vi "Teleop.vi"(10 "Match Info":T1={"Autonomous Elapsed Seconds"=0.0, "TeleOp Elapsed Seconds"=0.0, "Disabled Elapsed Seconds"=0.0, "Visited Autonomous"=FALSE, "Visited TeleOp"=FALSE, "Visited Disabled"=FALSE, "Autonomous Settings"={"Autonomous Style"=enum."Independent", "VI Refnum"=refnum}}, 11 "Call Context":T2) -> ()   [LabVIEW 2013]
doc: "This VI is called for each TeleOp packet received from the DS where the robot is not disabled. It is often used to read from the joysticks and update I/O or to update setpoints for timed control loops. It should complete and return within 20 milliseconds or it may miss DS packets."
uses:
  <vilib>/Rock Robotics/WPI/DriverStation/WPI_DriverStationDerivedRobotMode.ctl
  <vilib>/Rock Robotics/WPI/DriverStation/WPI_DriverStationMatch Info.ctl
  Robot Global Data.vi
  <vilib>/Rock Robotics/WPI/Joystick/WPI_JoystickGetSetRefNum.vi
panel:
  in  "HarvSpeed":dbl=0.5
  out "Distance 2":dbl
  out "Distance":dbl
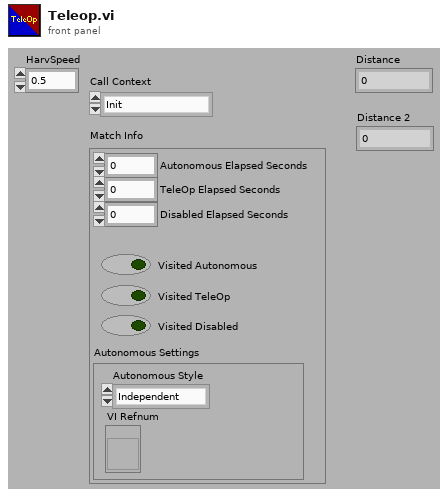
[diagram p1: front panel]
types:
  T1 = typedef "WPI_DriverStationMatch Info.ctl" = cluster{"Autonomous Elapsed Seconds":dbl, "TeleOp Elapsed Seconds":dbl, "Disabled Elapsed Seconds":dbl, "Visited Autonomous":bool, "Visited TeleOp":bool, "Visited Disabled":bool, "Autonomous Settings":cluster{"Autonomous Style":enum16{"Iterative", "Independent"}, "VI Refnum":refnum<vi>}}
  T2 = typedef "WPI_DriverStationDerivedRobotMode.ctl" = enum16{"Init", "Execute", "Stop"}
  T3 = typedef "WPI_JoystickDevRef.ctl" = cluster{"Device":T4}
  T4 = typedef "WPI_JoystickDeviceEnum.ctl" = enum16{"USB 1", "USB 2", "USB 3", "USB 4", "Kinect 1", "Kinect 2"}
  T5 = cluster{"axis 1 (x)":dbl, "axis 2 (y)":dbl, "axis 3 (throttle)":dbl, "axis 4":dbl, "axis 5":dbl, "axis 6":dbl}
  T6 = typedef "WPI_MotorControlDeviceRef.ctl" = cluster{"DeviceStatus":errorcluster, "Type":enum16{"PWM", "CAN"}, "PWM":cluster{"Digital Module":T7, "PWM Channel":T8, "DeadBand":T9}, "CAN":cluster{"Device Number":u8, "Control Mode":T10, "Semaphore":T11, "Max Vout":dbl}, "Invert":bool, "TransformRef":T12, "InvTransformRef":T12}
  T7 = typedef "FPGA_TypedefDigitalModule.ctl" = enum16{"Digital Module 1", "Digital Module 2"}
  T8 = typedef "FPGA_DIOPWMChannel.ctl" = enum8{"PWM 1", "PWM 2", "PWM 3", "PWM 4", "PWM 5", "PWM 6", "PWM 7", "PWM 8", "PWM 9", "PWM 10", "Invalid"}
  T9 = typedef "WPI_PWMDeadband.ctl" = cluster{"Name":string, "maxPositivePwm":i32, "minPositivePwm":i32, "centerPwm":i32, "maxNegativePwm":i32, "minNegativePwm":i32, "angularRange":u16}
  T10 = typedef "WPI_CANJaguar_ControlMode.ctl" = enum8{"Percent VBus", "Current", "Speed", "Position", "Voltage"}
  T11 = typedef "Semaphore RefNum" = refnum<k1>
  T12 = typedef "WPI_PWMTransform_ConPane.ctl" = refnum<vi>
  T13 = typedef "WPI_EncoderDevRef.ctl" = cluster{"DevStatus":errorcluster, "EncoderIndex":T14, "CounterIndex":T15, "DistancePerCount":dbl, "Decoding Type":T16}
  T14 = typedef "FPGA_EncoderIdx.ctl" = enum8{"Enc 0", "Enc 1", "Enc 2", "Enc 3", "Invalid"}
  T15 = typedef "FPGA_CounterCtrSystemIndex.ctl" = enum8{"Ctr 0", "Ctr 1", "Ctr 2", "Ctr 3", "Ctr 4", "Ctr 5", "Ctr 6", "Ctr 7", "Invalid"}
  T16 = typedef "WPI_EncoderType.ctl" = enum16{"1x", "2x", "4x"}
  T17 = typedef "WPI_JoystickButtonState.ctl" = cluster{"Button 1":bool, "Button 2":bool, "Button 3":bool, "Button 4":bool, "Button 5":bool, "Button 6":bool, "Button 7":bool, "Button 8":bool, "Button 9":bool, "Button 10":bool, "Button 11":bool, "Button 12":bool}
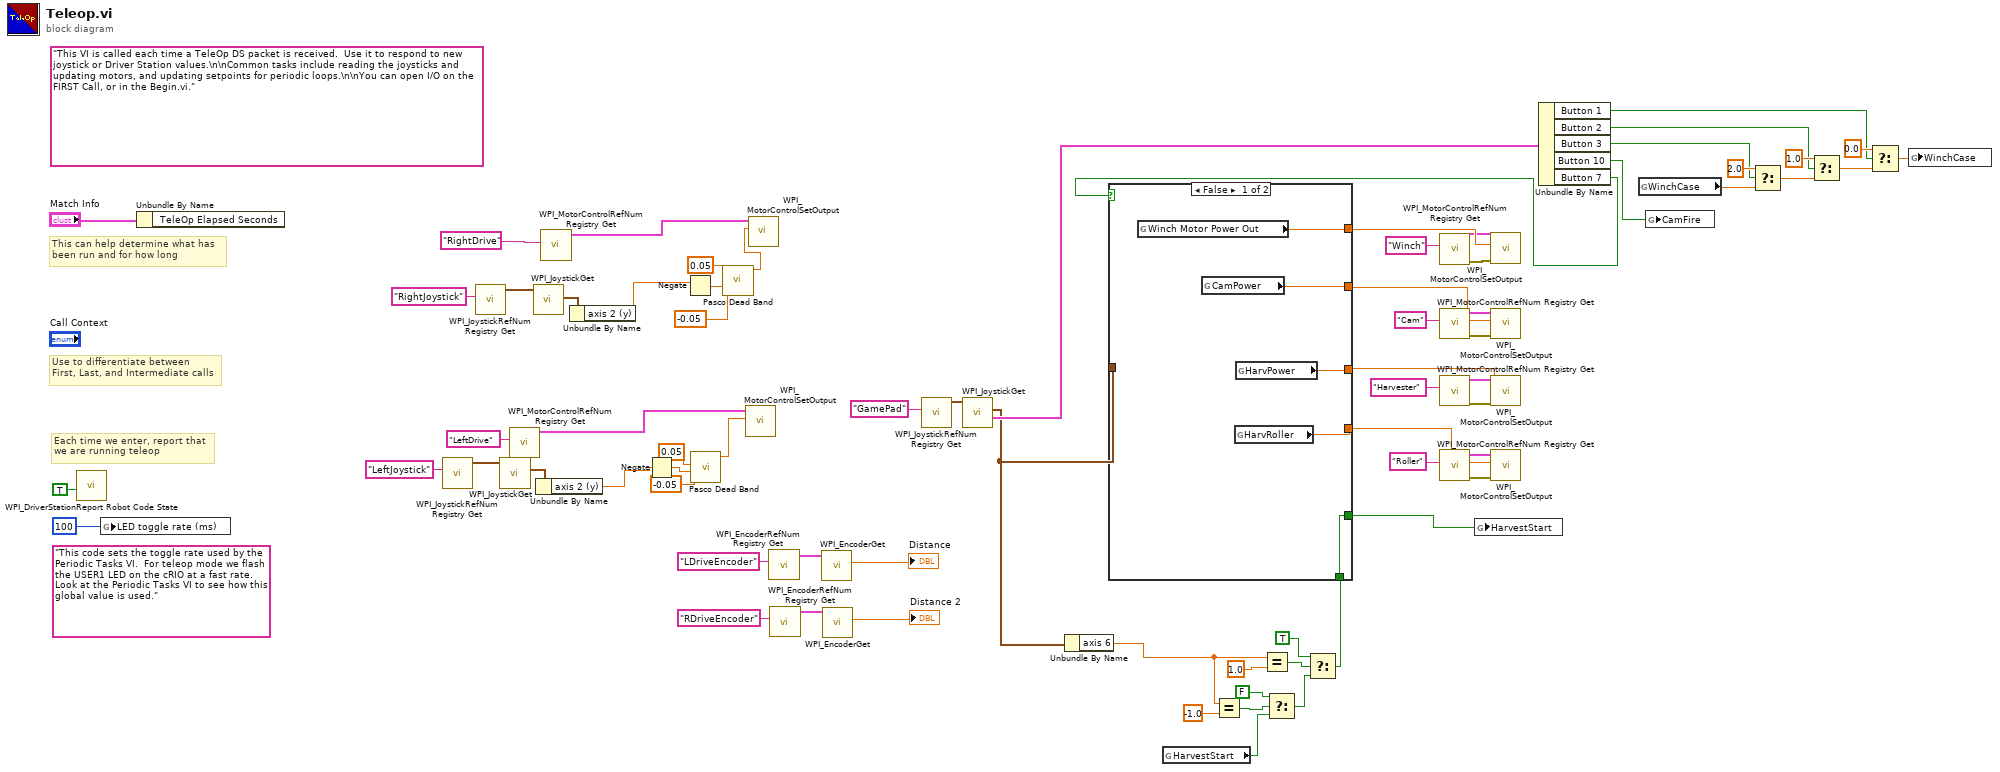
[diagram p0: block diagram]
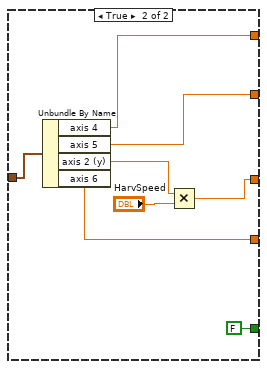
[diagram p2: hidden frame]
diagram:
  (unwired) "This code sets the toggle rate used by the Periodic Tasks VI.  For teleop mode we flash the USER1 LED on the cRIO at a fast rate.  Look at the Periodic Tasks VI to see how this global value is used."
  (unwired) "This VI is called each time a TeleOp DS packet is received.  Use it to respond to new joystick or Driver Station values.\n\nCommon tasks include reading the joysticks and updating motors, and updating setpoints for periodic loops.\n\nYou can open I/O on the FIRST Call, or in the Begin.vi."
  # "Each time we enter, report that\nwe are running teleop"
  # "Use to differentiate between\nFirst, Last, and Intermediate calls"
  # "This can help determine what has\nbeen run and for how long"
  n1 = call <vilib>:"WPI_DriverStationReport Robot Code State.vi"("TeleOp"=TRUE ("Autonomous")) -> ()  [unwired: 10 in, 1 out]
  n2 = global write "Robot Global Data.vi" "LED toggle rate (ms)"(u32 100 ("LED ms toggle rate")) -> ()
  n3 = Unbundle By Name("Match Info") -> ()  [unwired: 1 out]
  n4 = call <vilib>:"WPI_JoystickRefNum Registry Get.vi"("refnum name"="LeftJoystick") -> ("JoystickDevRef"=w61:T3)  [unwired: 9 in, 1 out]
  n5 = call <vilib>:"WPI_JoystickRefNum Registry Get.vi"("refnum name"="RightJoystick") -> ("JoystickDevRef"=w66:T3)  [unwired: 9 in, 1 out]
  n6 = call <vilib>:"WPI_JoystickGet.vi"("JoystickDevRef"=w61) -> ("Axes"=w60:T5)  [unwired: 4 in, 2 out]
  n7 = call <vilib>:"WPI_MotorControlRefNum Registry Get.vi"("refnum name"="LeftDrive") -> ("MotorControlDevRef"=w64:T6)  [unwired: 9 in, 1 out]
  n8 = call <vilib>:"WPI_JoystickGet.vi"("JoystickDevRef"=w66) -> ("Axes"=w65:T5)  [unwired: 4 in, 2 out]
  n9 = Unbundle By Name(w60) -> ("axis 2 (y)"=w59:dbl)
  n10 = call <vilib>:"WPI_MotorControlRefNum Registry Get.vi"("refnum name"="RightDrive") -> ("MotorControlDevRef"=w69:T6)  [unwired: 9 in, 1 out]
  n11 = Unbundle By Name(w65) -> ("axis 2 (y)"=w58:dbl)
  n12 = Negate(x=w59) -> (-x=w10:dbl)
  n13 = Negate(x=w58) -> (-x=w14:dbl)
  n14 = call "Pasco Dead Band.vi"("lower limit"=-0.05, "PWM Power"=w10, "upper limit"=0.05) -> ("PWM Power"=w7:dbl)  [unwired: 7 in, 1 out]
  n15 = call "Pasco Dead Band.vi"("lower limit"=-0.05, "PWM Power"=w14, "upper limit"=0.05) -> ("PWM Power"=w13:dbl)  [unwired: 7 in, 1 out]
  n16 = call <vilib>:"WPI_MotorControlSetOutput.vi"("Output"=w7, "MotorControlDevRef"=w64) -> ()  [unwired: 7 in, 3 out]
  n17 = call <vilib>:"WPI_MotorControlSetOutput.vi"("Output"=w13, "MotorControlDevRef"=w69) -> ()  [unwired: 7 in, 3 out]
  n18 = call <vilib>:"WPI_EncoderRefNum Registry Get.vi"("refnum name"="LDriveEncoder") -> ("EncoderDevRef"=w26:T13)  [unwired: 9 in, 1 out]
  n19 = call <vilib>:"WPI_EncoderRefNum Registry Get.vi"("refnum name"="RDriveEncoder") -> ("EncoderDevRef"=w5:T13)  [unwired: 9 in, 1 out]
  n20 = call <vilib>:"WPI_EncoderGet.vi"("EncoderDevRef"=w26) -> ("Distance"=→"Distance":dbl)  [unwired: 5 in, 5 out]
  n21 = call <vilib>:"WPI_EncoderGet.vi"("EncoderDevRef"=w5) -> ("Distance"=→"Distance 2":dbl)  [unwired: 5 in, 5 out]
  n22 = call <vilib>:"WPI_JoystickRefNum Registry Get.vi"("refnum name"="GamePad") -> ("JoystickDevRef"=w56:T3)  [unwired: 9 in, 1 out]
  n23 = call <vilib>:"WPI_JoystickGet.vi"("JoystickDevRef"=w56) -> ("Buttons"=w29:T17, "Axes"=w24:T5)  [unwired: 4 in, 1 out]
  n24 = Unbundle By Name(w24) -> ("axis 6"=w16:dbl)
  n25 = global read "Robot Global Data.vi" "HarvestStart"() -> (w15:bool)
  n26 = Equal?(x=w16, y=-1.0) -> (x = y?=w17:bool)
  n27 = Equal?(x=w16, y=1.0) -> (x = y?=w22:bool)
  n28 = Select(t=FALSE, s=w17, f=w15) -> (s? t:f=w19:bool)
  n29 = Select(t=TRUE, s=w22, f=w19) -> (s? t:f=w3:bool)
  n30 = call <vilib>:"WPI_MotorControlRefNum Registry Get.vi"("refnum name"="Winch") -> ("error out"=w47:errorcluster, "MotorControlDevRef"=w41:T6)  [unwired: 9 in]
  n31 = call <vilib>:"WPI_MotorControlRefNum Registry Get.vi"("refnum name"="Cam") -> ("error out"=w46:errorcluster, "MotorControlDevRef"=w45:T6)  [unwired: 9 in]
  n32 = call <vilib>:"WPI_MotorControlRefNum Registry Get.vi"("refnum name"="Harvester") -> ("error out"=w51:errorcluster, "MotorControlDevRef"=w50:T6)  [unwired: 9 in]
  n33 = call <vilib>:"WPI_MotorControlRefNum Registry Get.vi"("refnum name"="Roller") -> ("error out"=w53:errorcluster, "MotorControlDevRef"=w54:T6)  [unwired: 9 in]
  n34 = Unbundle By Name(w29) -> ("Button 1"=w32:bool, "Button 2"=w33:bool, "Button 3"=w34:bool, "Button 10"=w28:bool, "Button 7"=w1:bool)
  n35 = case shown="False" w1 {
    tunnel: [w77 w84] -> w52
    tunnel: [w76 w79] -> w48
    tunnel: w24 -> [_ w85]
    tunnel: [w74 w83] -> w42
    tunnel: [w75 w82] -> w40
    tunnel: w3 -> [w73 _]
    tunnel: [w73 FALSE ("HarvestStart")] -> w2
    frame False {
      n36 = global read "Robot Global Data.vi" "Winch Motor Power Out"() -> (w74:dbl)
      n37 = global read "Robot Global Data.vi" "CamPower"() -> (w75:dbl)
      n38 = global read "Robot Global Data.vi" "HarvRoller"() -> (w77:dbl)
      n39 = global read "Robot Global Data.vi" "HarvPower"() -> (w76:dbl)
    }
    frame True {
      n40 = Unbundle By Name(w85) -> ("axis 4"=w83:dbl, "axis 5"=w82:dbl, "axis 2 (y)"=w80:dbl, "axis 6"=w84:dbl)
      n41 = Multiply(x=w80, y="HarvSpeed") -> (x*y=w79:dbl)
    }
  }
  n42 = global write "Robot Global Data.vi" "HarvestStart"(w2) -> ()
  n43 = call <vilib>:"WPI_MotorControlSetOutput.vi"("error in (no error)"=w47, "Output"=w42, "MotorControlDevRef"=w41) -> ()  [unwired: 6 in, 3 out]
  n44 = call <vilib>:"WPI_MotorControlSetOutput.vi"("error in (no error)"=w46, "Output"=w40, "MotorControlDevRef"=w45) -> ()  [unwired: 6 in, 3 out]
  n45 = call <vilib>:"WPI_MotorControlSetOutput.vi"("error in (no error)"=w51, "Output"=w48, "MotorControlDevRef"=w50) -> ()  [unwired: 6 in, 3 out]
  n46 = call <vilib>:"WPI_MotorControlSetOutput.vi"("error in (no error)"=w53, "Output"=w52, "MotorControlDevRef"=w54) -> ()  [unwired: 6 in, 3 out]
  n47 = global read "Robot Global Data.vi" "WinchCase"() -> (w30:dbl)
  n48 = global write "Robot Global Data.vi" "CamFire"(w28) -> ()
  n49 = Select(t=2.0, s=w34, f=w30) -> (s? t:f=w39:dbl)
  n50 = Select(t=1.0, s=w33, f=w39) -> (s? t:f=w38:dbl)
  n51 = Select(t=0.0, s=w32, f=w38) -> (s? t:f=w31:dbl)
  n52 = global write "Robot Global Data.vi" "WinchCase"(w31) -> ()
